vi "Get Build.vi"(8 "error in (no error)":errorcluster, 9 "index":i32, 11 "Builder in":refnum<class "Builder.lvclass">) -> (0 "error out":errorcluster, 2 "build modified":T1={"App Name"="", "Build Type"=enum."Build", "Current Version"="", "Next Version"="", "Check"=FALSE}, 3 "Builder out":refnum<class "Builder.lvclass">)   [LabVIEW 2021, in "App-Builder Library.lvlib" / "Builder.lvclass"]
uses:
  Builder.lvclass
  Build Type.ctl
  App descriptions.ctl
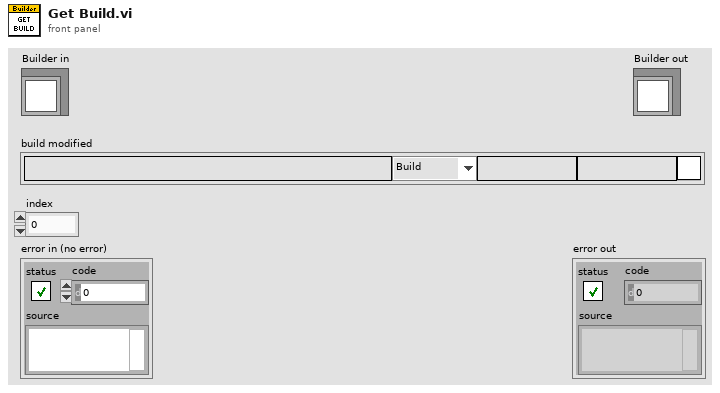
[diagram p1: front panel]
types:
  T1 = typedef "App-Builder Library.lvlib/Builder.lvclass/App descriptions.ctl" = cluster{"App Name":string, "Build Type":T2, "Current Version":string, "Next Version":string, "Check":bool}
  T2 = typedef "App-Builder Library.lvlib/Builder.lvclass/Build Type.ctl" = enum16{"Major", "Minor", "Fix", "Build"}
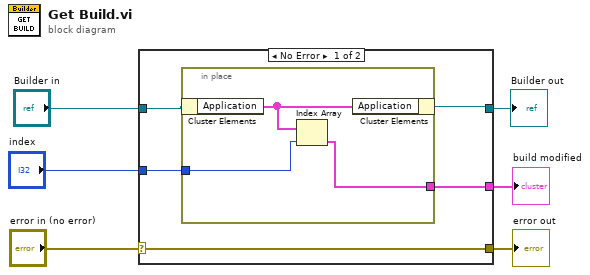
[diagram p0: block diagram]
diagram:
  n1 = case shown="No Error" "error in (no error)" {
    selector: "error in (no error)" -> [w11 w16]
    tunnel: [w11 w16] -> w5
    tunnel: [w9 w15] -> w3
    tunnel: "Builder in" -> [w10 w15]
    tunnel: [w8 _] -> w1
    tunnel: "index" -> [w7 _]
    frame No Error {
      n2 = in-place {
        in-place-border: w7 -> [w12]
        in-place-border: [w13] -> w8
        n3 = in-place-cluster #1(w10) -> ("Application"=w14:T1[])
        n4 = Index Array(array=w14, index=w12) -> (element=w13:T1)
        n5 = in-place-cluster #1("Application"=w14) -> (w9:refnum<class "Builder.lvclass">)
      }
    }
    frame Error {
    }
  }
  "error out" <- w5
  "Builder out" <- w3
  "build modified" <- w1
